vi "AIP Parser.vi"(8 "error in (no error)":errorcluster, 10 "RDS Serial Frame":refnum<class "RDS Serial Frame.lvclass">, 11 "AIP Instrument in":refnum<class "AIP Instrument.lvclass">) -> (0 "error out":errorcluster, 2 "AIP Status Response":refnum<class "AIP Status Response.lvclass">, 3 "AIP Instrument out":refnum<class "AIP Instrument.lvclass">)   [LabVIEW 2015, in "AIP Instrument.lvlib" / "AIP Instrument.lvclass"]
uses:
  AIP Instrument.lvclass
  Libraries/RDS Serial Handler/RDS Serial Frame.lvclass
  Libraries/RDS Child Messages/AIP Status Message/AIP Status Response.lvclass
  Libraries/RDS Instruments/AIP/AIP Status.ctl
  Libraries/RDS Instruments/AIP/AIP States.ctl
  Libraries/RDS Serial Handler/RDS Serial Frame.lvclass/RDS Serial Frame.ctl
  Libraries/RDS Framework/RDS Message ID.ctl
  Libraries/RDS Framework/RDS Message Class/RDS Message.lvclass/RDS Message.ctl
  AIP Instrument.lvclass/AIP Instrument.ctl
  Libraries/RDS Child Messages/AIP Status Message/AIP Status Response.lvclass/AIP Status Response.ctl
  Libraries/RDS Instruments/RDS Instrument Library.lvlib
  Libraries/RDS Child Messages/RDS Child Messages.lvlib
  Libraries/RDS Framework/RDS Message Class/RDS Message.lvclass
  Libraries/RDS Serial Handler/RDS Serial Handler.lvlib
panel:
  out "AIP State":T1
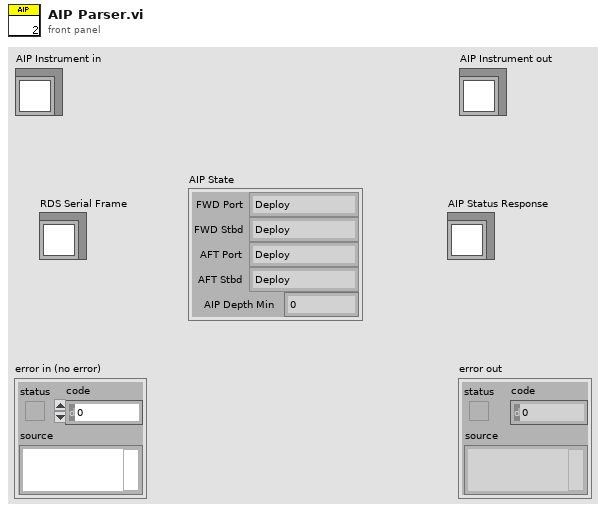
[diagram p1: front panel]
types:
  T1 = typedef "RDS Instrument Library.lvlib/AIP Status.ctl" = cluster{"FWD Port":T2, "FWD Stbd":T2, "AFT Port":T2, "AFT Stbd":T2, "AIP Depth Min":u8}
  T2 = typedef "RDS Instrument Library.lvlib/AIP States.ctl" = enum16{"Deploy", "Deploying", "Deployed", "Stow", "Stowing", "Stowed", "Fault", "brakeOnStow", "breakOnDeploy", "Stopped", "Stopping"}
  T3 = typedef "RDS Child Messages.lvlib/RDS Message ID.ctl" = enum16{"RDS Hello World", "String Message", "AIP_Status", "AIP_Command", "GPS_Data", "MCB_Command", "MCB_Status", "Compass_Data", "Depth_Data", "Battery_Data", "Contoller_State", "Set_Mag_Dev", "BTB_Shutdown", "State_Sample_Request", "State_Sample", "PID_Gains_Set", "Helm_Limiter_Set", "Helm_Heading_Command", "Helm_Steering_Command", "Helm_Status", "Controller_Message", "AIP_Set_Min_Depth", "Mission_Controller_State", "Mission_Upload", "Mission_Set_Op_and_Run", "Mission_Settings_Set"}
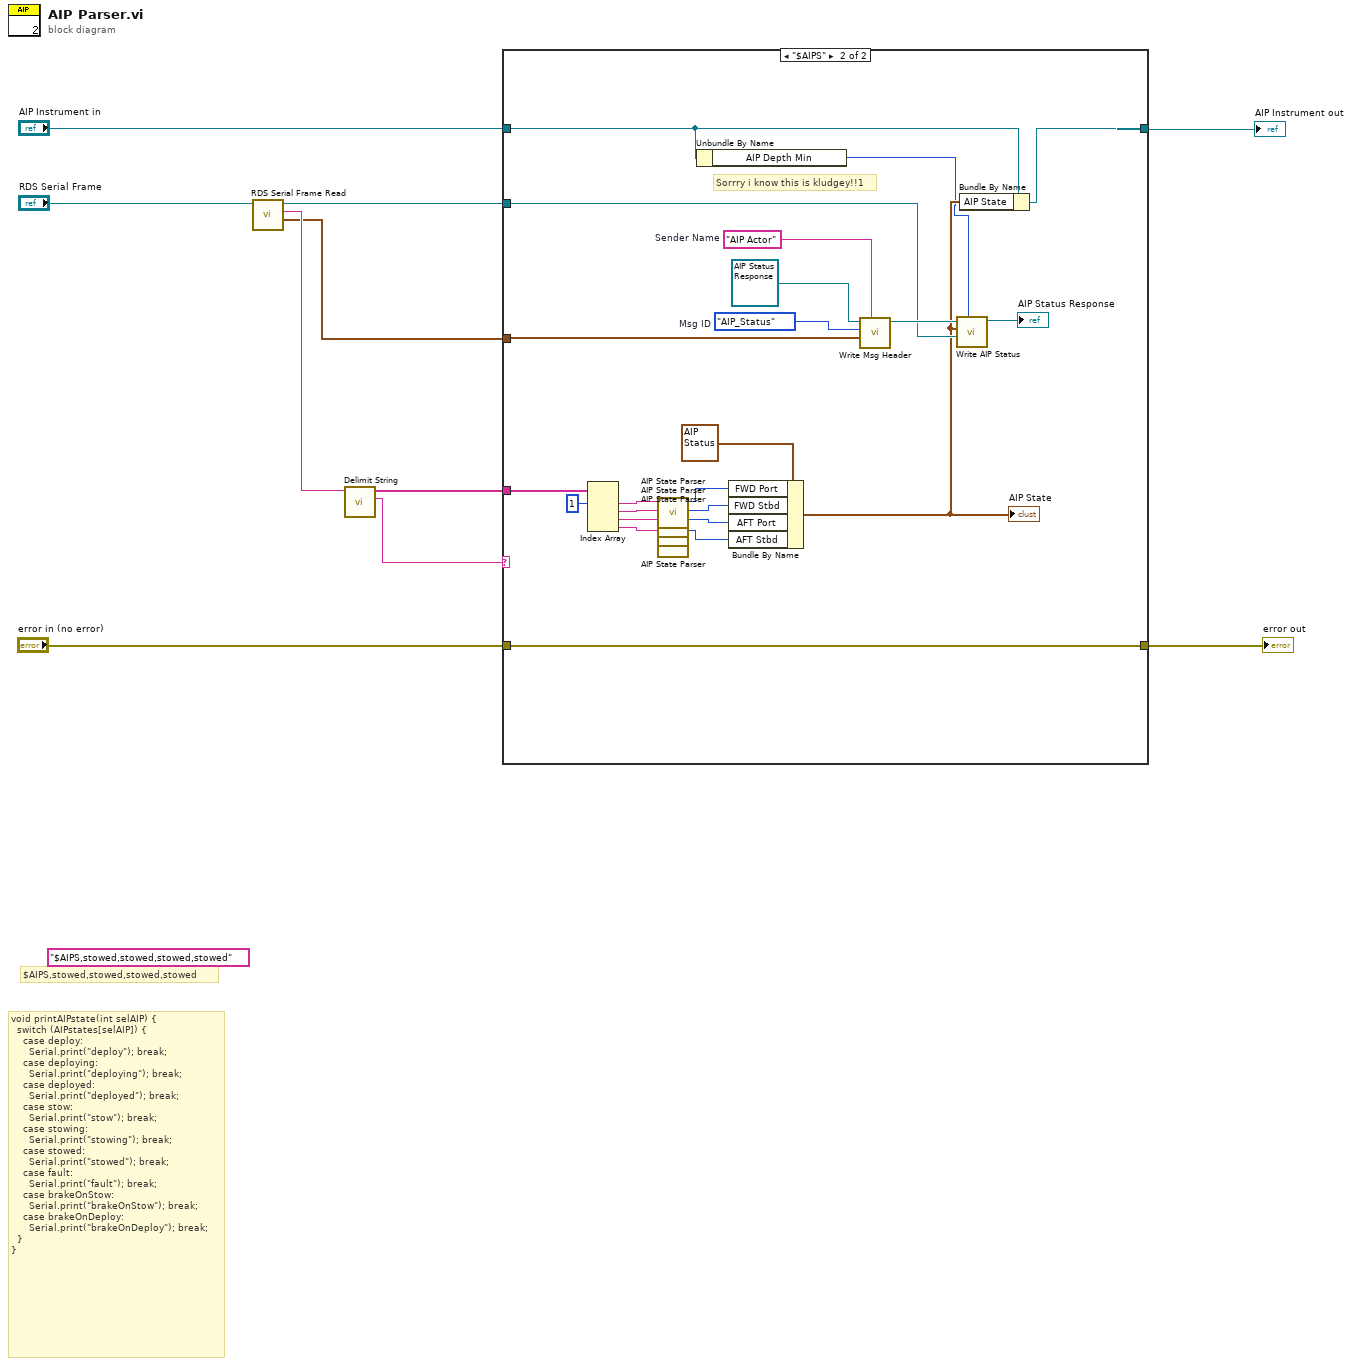
[diagram p0: block diagram]
diagram:
  (unwired) "$AIPS,stowed,stowed,stowed,stowed"
  # "void printAIPstate(int selAIP) {\n  switch (AIPstates[selAIP]) {\n    case deploy:\n      Serial.print(\"deploy\"); break;\n    case deploying:\n      Serial.print(\"deploying\"); break;\n    case deployed:\n      Serial.print(\"deployed\"); break;\n    case stow:\n      Serial.print(\"stow\"); break;\n    case stowing:\n      Serial.print(\"stowing\"); break;\n    case stowed:\n      Serial.print(\"stowed\"); break;\n    case fault:\n      Serial.print(\"fault\"); break;\n    case brakeOnStow:\n      Serial.print(\"brakeOnStow\"); break;\n    case brakeOnDeploy:\n      Serial.print(\"brakeOnDeploy\"); break;\n  }\n}"
  # "$AIPS,stowed,stowed,stowed,stowed"
  n1 = call "RDS Serial Frame Read.vi"("RDS Serial Frame in"="RDS Serial Frame") -> ("Time Stamp"=w6:timestamp, "Serial String"=w7:string, "RDS Serial Frame out"=w5:refnum<class "RDS Serial Frame.lvclass">)  [unwired: 7 in, 1 out]
  n2 = call "Delimit String.vi"("Serial String"=w7) -> ("First Element"=w8:string, "All Elements"=w9:string[])  [unwired: 9 in]
  n3 = case shown="\"$AIPS\"" w8 {
    tunnel: w9 -> [_ w35]
    tunnel: w6 -> [_ w23]
    tunnel: w5 -> [_ w19]
    tunnel: [w12 w15] -> w3
    tunnel: "AIP Instrument in" -> [w12 w14]
    tunnel: [w11 w17] -> w2
    tunnel: "error in (no error)" -> [w11 w17]
    frame "False", Default {
    }
    frame "$AIPS" {
      w21 = "AIP Actor"  # Sender Name
      w22 = RDS_Message_ID."AIP_Status"  # Msg ID
      # "Sorrry i know this is kludgey!!1"
      n4 = Index Array(array=w35, index #1=1 ("index")) -> (element #1=w34:string, element #2=w33:string, element #3=w32:string, element #4=w31:string)  [unwired: 3 in]
      n5 = call "AIP State Parser.vi"("String"=w34) -> ("AIP States"=w29:T2)  [unwired: 8 in]
      n6 = call "AIP State Parser.vi"("String"=w33) -> ("AIP States"=w28:T2)  [unwired: 8 in]
      n7 = call "AIP State Parser.vi"("String"=w32) -> ("AIP States"=w27:T2)  [unwired: 8 in]
      n8 = call "AIP State Parser.vi"("String"=w31) -> ("AIP States"=w26:T2)  [unwired: 8 in]
      n9 = Unbundle By Name(w14) -> ("AIP Depth Min"=w13:u8)
      n10 = Bundle By Name(cluster=T1 {"FWD Port"=enum."Deploy", "FWD Stbd"=enum."Deploy", "AFT Port"=enum."Deploy", "AFT Stbd"=enum."Deploy", "AIP Depth Min"=0} ("AIP Status"), "FWD Port"=w29, "FWD Stbd"=w28, "AFT Port"=w27, "AFT Stbd"=w26) -> (w16:T1)
      "AIP State" <- w16
      n11 = call "Write Msg Header.vi"("Sender Name"=w21, "Time Stamp"=w23, "Msg ID"=w22, "RDS Message in"=refnum<class "AIP Status Response.lvclass"> refnum ("RDS Child Messages.lvlib:AIP Status Response.lvclass")) -> ("RDS Message out"=w20:refnum<class "AIP Status Response.lvclass">)  [unwired: 6 in, 1 out]
      n12 = call "Write AIP Status.vi"("AIP Depth Min"=w13, "Raw Frame"=w19, "AIP Status"=w16, "AIP Status Response in"=w20) -> ("AIP Status Response out"=→"AIP Status Response":refnum<class "AIP Status Response.lvclass">)  [unwired: 6 in, 1 out]
      n13 = Bundle By Name(cluster=w14, "AIP State"=w16) -> (w15:refnum<class "AIP Instrument.lvclass">)
    }
  }
  "error out" <- w2
  "AIP Instrument out" <- w3
